vi "Clear Buffers (No Objects, Anritsu).vi"(8 "error in (no error)":errorcluster, 11 "Cluster In":T13={"Channel Names"=[], "Channel Units"=[], "Most Recent Data Points"=[], "History Buffers"=[], "Ring Buffers"=[], "Averaging"=enum."On", "Units"=enum."Watt", "Measuring rate"=enum."Hold", "Unit Range"=enum."10 mW (+10 dBm)", "Calibration Factor"=-26.67, "Auto Ranging?"=enum."Off"}) -> (0 "error out":errorcluster, 3 "Cluster Out":T13={"Channel Names"=[], "Channel Units"=[], "Most Recent Data Points"=[], "History Buffers"=[], "Ring Buffers"=[], "Averaging"=enum."On", "Units"=enum."Watt", "Measuring rate"=enum."Hold", "Unit Range"=enum."10 mW (+10 dBm)", "Calibration Factor"=-26.67, "Auto Ranging?"=enum."Off"})   [LabVIEW 2009]
uses:
  Channel Names.ctl
  Channel Units.ctl
  Data Points.ctl
  Data Point.ctl
  Time.ctl
  X.ctl
  TX Graph.ctl
  Anritsu Power Meter/Anritsu Power Meter/Public/Averaging control.ctl
  Anritsu Power Meter/Anritsu Power Meter/Public/Display control.ctl
  Anritsu Power Meter/Anritsu Power Meter/Public/Measuring rate control.ctl
  Anritsu Power Meter/Anritsu Power Meter/Public/Range control watts and dBm.ctl
  Anritsu Power Meter/Anritsu Power Meter/Public/Auto Range control.ctl
  Readable.lvclass
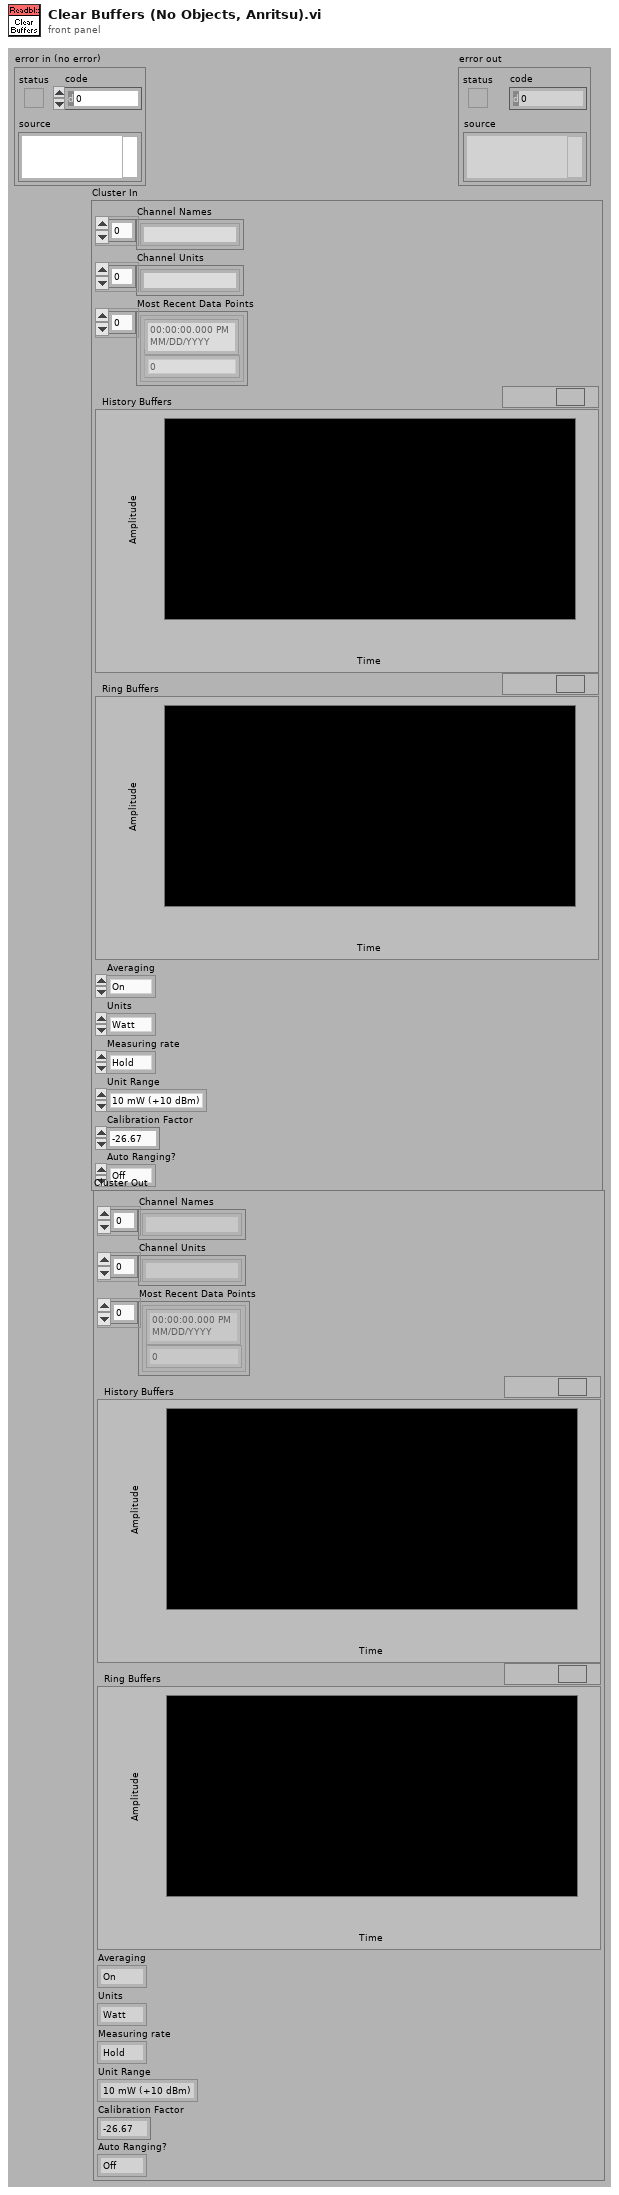
[diagram p1: front panel]
types:
  T1 = typedef "Readable.lvclass/Channel Names.ctl" = string[]
  T2 = typedef "Readable.lvclass/Channel Units.ctl" = string[]
  T3 = typedef "Readable.lvclass/Data Points.ctl" = T4[]
  T4 = typedef "Readable.lvclass/Data Point.ctl" = cluster{"t":T5, "x":T6}
  T5 = typedef "Readable.lvclass/Time.ctl" = timestamp
  T6 = typedef "Readable.lvclass/X.ctl" = dbl
  T7 = typedef "Readable.lvclass/TX Graph.ctl" = cluster{"Data Points":cluster{"t":timestamp, "x":dbl}[]}[]
  T8 = typedef "Averaging control.ctl" = enum16{"On", "Off"}
  T9 = typedef "Display control.ctl" = enum16{"Watt", "dBm", "dB (REL)"}
  T10 = typedef "Measuring rate control.ctl" = enum16{"Hold", "Free Run", "Exit Trigger"}
  T11 = typedef "Range control watts and dBm.ctl" = enum16{"10 mW (+10 dBm)", "1 mW (0 dBm)", "100 uW (-10 dBm)", "10 uW (-20 dBm)", "1 uW (-30 dBm)", "100 nW (-40 dBm)", "10 nW (-50 dBm)", "1 nW (-60 dBm)", "100 pW (-70 dBm)", "10 pW (-80 dBm)"}
  T12 = typedef "Auto Range control.ctl" = enum16{"Off", "On"}
  T13 = cluster{"Channel Names":T1, "Channel Units":T2, "Most Recent Data Points":T3, "History Buffers":T7, "Ring Buffers":T7, "Averaging":T8, "Units":T9, "Measuring rate":T10, "Unit Range":T11, "Calibration Factor":dbl, "Auto Ranging?":T12}
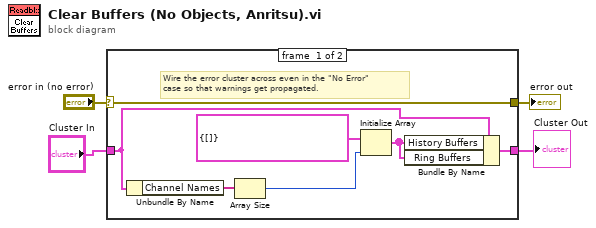
[diagram p0: block diagram]
diagram:
  n1 = case shown="No Error" "error in (no error)" {
    selector: "error in (no error)" -> [w11 w13]
    tunnel: [w11 w13] -> w3
    tunnel: [w9 w12] -> w1
    tunnel: "Cluster In" -> [w7 w12]
    frame #0 {
      # "Wire the error cluster across even in the \"No Error\"\ncase so that warnings get propagated."
      n2 = Unbundle By Name(w7) -> ("Channel Names"=w6:T1)
      n3 = Array Size(array=w6) -> (size(s)=w5:i32)
      n4 = Initialize Array(cluster{T4[]} {[]} ("output cluster"), w5) -> (w8:cluster{T4[]}[])
      n5 = Bundle By Name(cluster=w7, "History Buffers"=w8, "Ring Buffers"=w8) -> (w9:T13)
    }
    frame #1 {
    }
  }
  "error out" <- w3
  "Cluster Out" <- w1
